vi "Database.vi"() -> ()   [LabVIEW 2017]
uses:
  D:/source/VI/JAC_Database/JAC_DataBase.dll
  JAC_DataBase.dll
panel:
  in  "筛选页数":i32=1 caption="页数" min=1 max=1 step=1 format="%.0f/1"
  in  "每页数量":i32
  in  "筛选按钮":bool
  in  "筛选值（支持模糊筛选）":string
  in  "表字段下拉菜单":u16(ring) caption="选择筛选字段"
  in  "表名下拉菜单":u16(ring) caption="选择数据表" items=["请选择...", "四轮定位工位配置", "大灯工位配置", "侧滑工位配置", "制动工位配置", "车辆信息表"]
  in  "删除按钮":bool
  in  "刷新按钮":bool caption="刷新显示"
  in  "修改按钮":bool caption="修改数据库"
  in  "页数":i32=1 min=0 max=1 step=1 format="%.0f/0"
  in  "停止按钮":bool
  in  "记录表格":string[][](table) caption="查询记录"
  # "说明：\n1、表记录的列首为数据库字段名，不可更改。\n2、表记录的行首为记录ID号，也不可更改。\n3、修改数据库以选择行（红色框）为修改范围，\n     选择有ID的记录为更新，无ID的记录为插入。\n4、删除记录，以选择行（红色框）为删除范围。"
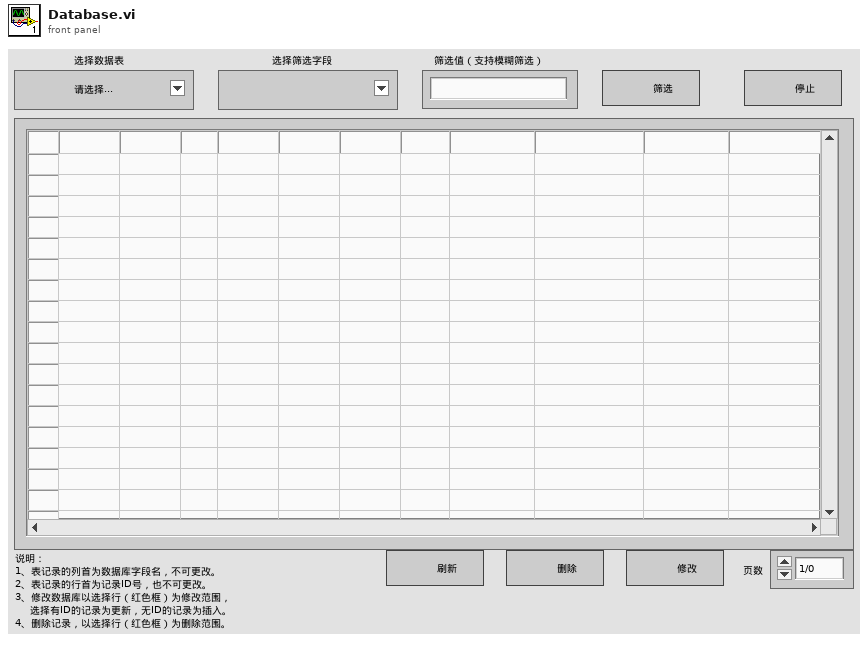
[diagram p1: front panel]
types:
  T1 = typedef "LVRowAndColumnTypeDef.ctl" = cluster{"Row":i32, "Column":i32}
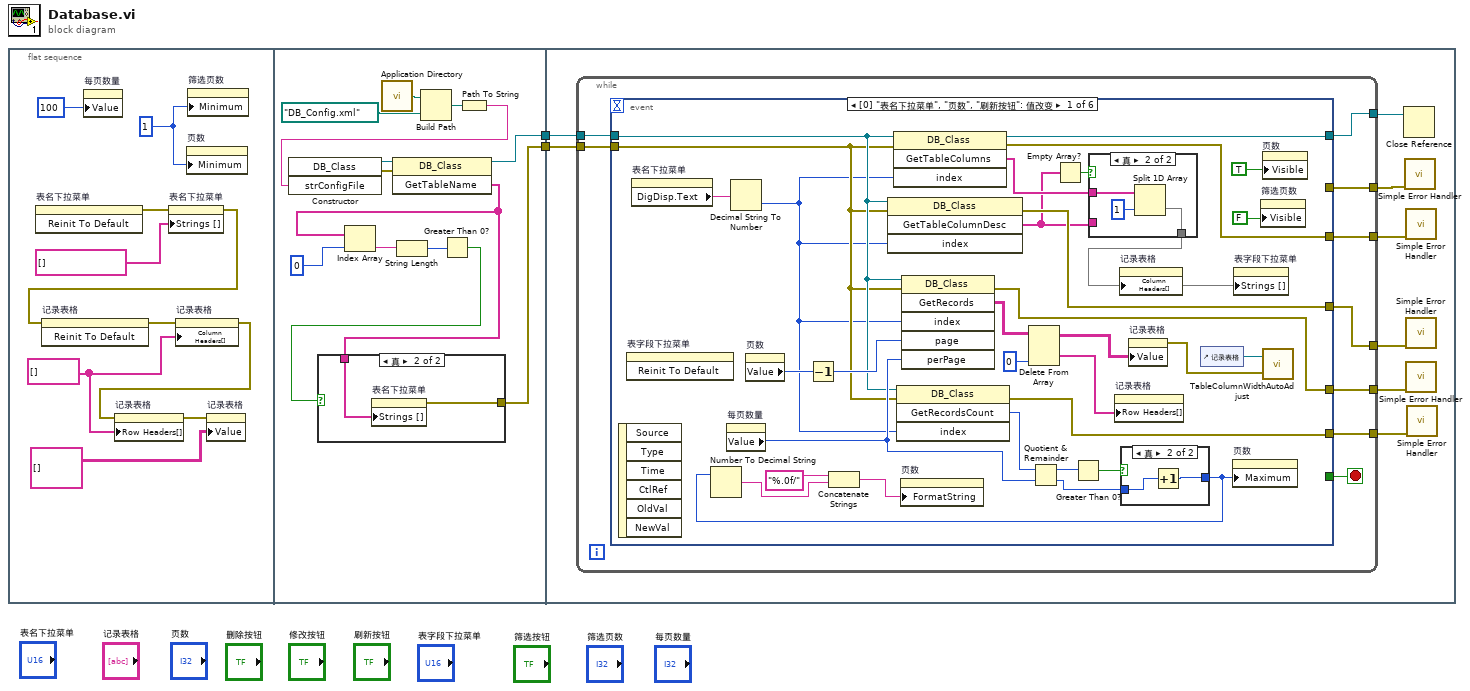
[diagram p0: block diagram]
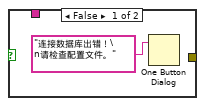
[diagram p2: hidden frame]
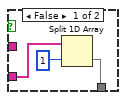
[diagram p3: hidden frame]
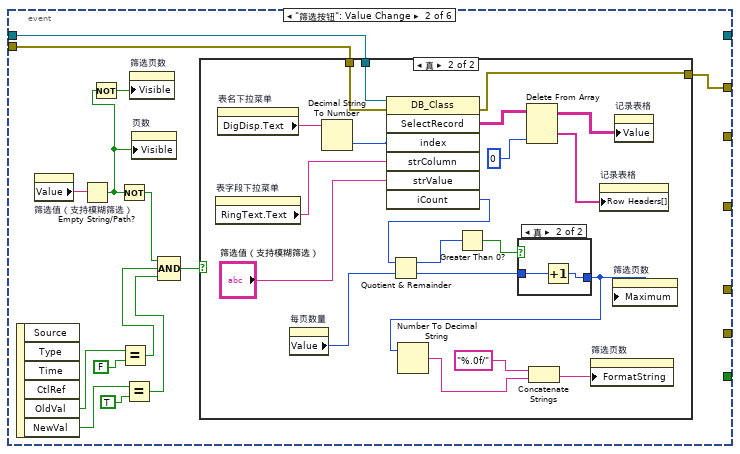
[diagram p5: hidden frame]
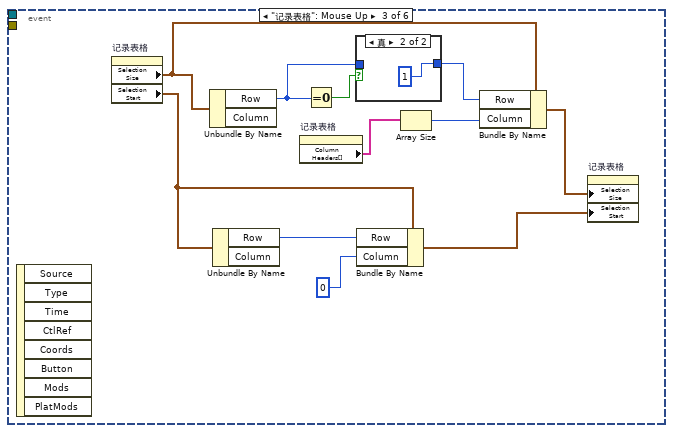
[diagram p8: hidden frame]
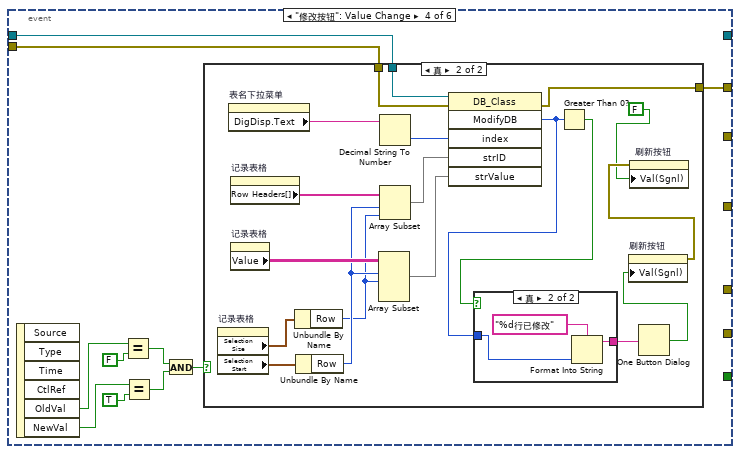
[diagram p10: hidden frame]
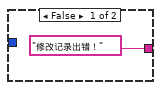
[diagram p12: hidden frame]
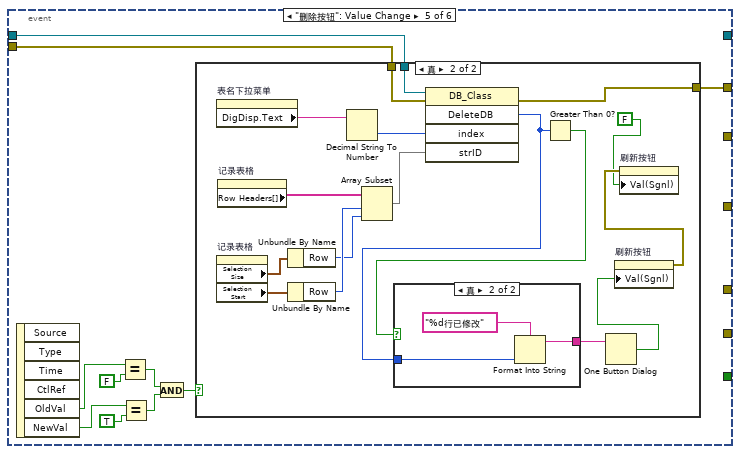
[diagram p13: hidden frame]
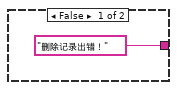
[diagram p15: hidden frame]
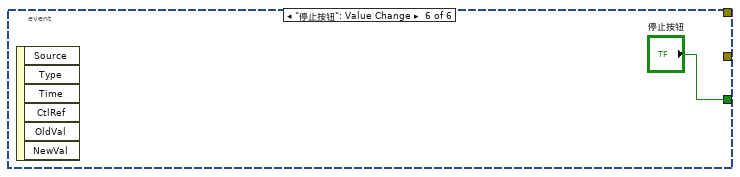
[diagram p16: hidden frame]
diagram:
  n1 = flat-sequence {
    tunnel: [w14] -> w2
    tunnel: [w13] -> w1
    tunnel: w2 -> [w33]
    tunnel: w1 -> [w32]
    frame #0 {
      w3 = 1
      w7 = string[] []
      n2 = invoke on="表名下拉菜单" class="Ring (严格)" method="Reinit To Default"() -> (error out=w12:errorcluster)  [unwired: 3 in, 2 out]
      n3 = property on="每页数量" class="DigNum (严格)"("Value"=100) -> ()  [unwired: 2 in, 2 out]
      n4 = property on="表名下拉菜单" class="Ring (严格)"(error in=w12, "Strings []"=string[] []) -> (error out=w10:errorcluster)  [unwired: 1 in, 1 out]
      n5 = invoke on="记录表格" class="Tbl (严格)" method="Reinit To Default"(error in=w10) -> (error out=w9:errorcluster)  [unwired: 2 in, 2 out]
      n6 = property on="记录表格" class="Tbl (严格)"(error in=w9, "Column Headers[]"=w7) -> (error out=w8:errorcluster)  [unwired: 1 in, 1 out]
      n7 = property on="记录表格" class="Tbl (严格)"(error in=w8, "Row Headers[]"=w7) -> (error out=w6:errorcluster)  [unwired: 1 in, 1 out]
      n8 = property on="页数" class="DigNum (严格)"("Minimum"=w3) -> ()  [unwired: 2 in, 2 out]
      n9 = property on="筛选页数" class="DigNum (严格)"("Minimum"=w3) -> ()  [unwired: 2 in, 2 out]
      n10 = property on="记录表格" class="Tbl (严格)"(error in=w6, "Value"=string[][] []) -> ()  [unwired: 1 in, 2 out]
    }
    frame #1 {
      n11 = call <vilib>:"Application Directory.vi"() -> ("Application Directory"=w17:path)
      n12 = Build Path(base path=w17, name or relative path=path "DB_Config.xml") -> (appended path=w18:path)
      n13 = Path To String(path=w18) -> (string=w19:string)
      n14 = constructor class="DB_Class"("strConfigFile"=w19) -> (reference out=w20:refnum<k24>, error out=w21:errorcluster)  [unwired: 3 in, 2 out]
      n15 = invoke on="调用节点" class="DB_Class" method="GetTableName"(reference=w20, error in=w21) -> (reference out=w14:refnum<k24>, "GetTableName"=w25:string[])  [unwired: 1 in, 1 out]
      n16 = Index Array(array=w25, index=0) -> (element=w22:string)
      n17 = String Length(string=w22) -> (length=w23:i32)
      n18 = Greater Than 0?(x=w23) -> (x > 0?=w24:bool)
      n19 = case shown="真" w24 {
        tunnel: w25 -> [_ w28]
        tunnel: [_ w27] -> w13
        frame False {
          n20 = One Button Dialog(message="连接数据库出错！\n请检查配置文件。") -> ()  [unwired: 1 in, 1 out]
        }
        frame True {
          n21 = property on="表名下拉菜单" class="Ring (严格)"("Strings []"=w28) -> (error out=w27:errorcluster)  [unwired: 2 in, 1 out]
        }
      }
    }
    frame #2 {
      n22 = while {
        tunnel: [w44] -> w36
        tunnel: [w43] -> w35
        tunnel: [w42] -> w34
        tunnel: w33 -> [w41]
        tunnel: w32 -> [w40]
        tunnel: [w39] -> w31
        tunnel: [w38] -> w30
        tunnel: [w37] -> w29
        stop <- w45 stop-if-true
        n23 = event shown="[0] \"表名下拉菜单\", \"页数\", \"刷新按钮\": 值改变" {
          selector: _ -> [_ _ _ _ _ _]
          dyn-events: _ -> [_ _ _ _ _ _]
          timeout: _ -> [_ _ _ _ _ _]
          tunnel: [_ _ _ _ _ "停止按钮"] -> w45
          tunnel: w41 -> [w56 w96 _ w140 w172 _]
          tunnel: w40 -> [w55 w95 _ w139 w171 _]
          tunnel: [w73 _ _ _ _ _] -> w44
          tunnel: [w72 _ _ _ _ _] -> w43
          tunnel: [_ w94 _ w138 w170 _] -> w42
          tunnel: [w71 _ _ _ _ _] -> w39
          tunnel: [w61 _ _ _ _ _] -> w38
          tunnel: [w52 _ _ _ _ _] -> w37
          event "表名下拉菜单", "页数", "刷新按钮": Value Change {
            n24 = event-data() -> ()  [unwired: 1 in, 6 out]
            n25 = invoke on="表字段下拉菜单" class="Ring (严格)" method="Reinit To Default"() -> ()  [unwired: 3 in, 3 out]
            n26 = property on="表名下拉菜单" class="Ring (严格)"() -> ("DigDisp.Text"=w49:string)  [unwired: 2 in, 2 out]
            n27 = property on="每页数量" class="DigNum (严格)"() -> ("Value"=w57:i32)  [unwired: 2 in, 2 out]
            n28 = Decimal String To Number(string=w49) -> (number=w48:i32)  [unwired: 2 in, 1 out]
            n29 = property on="页数" class="DigNum (严格)"() -> ("Value"=w58:i32)  [unwired: 2 in, 2 out]
            n30 = Decrement(x=w58) -> (x-1=w77:i32)
            n31 = invoke on="调用节点" class="DB_Class" method="GetTableColumnDesc"(reference=w56, error in=w55, "index"=w48) -> (error out=w52:errorcluster, "GetTableColumnDesc"=w51:string[])  [unwired: 1 in, 2 out]
            n32 = invoke class="DB_Class" method="GetTableColumns"(reference=w56, error in=w55, "index"=w48) -> (reference out=w61:refnum<k24>, error out=w73:errorcluster, "GetTableColumns"=w53:string[])  [unwired: 1 in, 1 out]
            n33 = invoke on="调用节点" class="DB_Class" method="GetRecordsCount"(reference=w56, error in=w55, "index"=w48) -> (error out=w71:errorcluster, "GetRecordsCount"=w67:i32)  [unwired: 1 in, 2 out]
            n34 = invoke class="DB_Class" method="GetRecords"(reference=w56, error in=w55, "index"=w48, "page"=w77, "perPage"=w57) -> (error out=w72:errorcluster, "GetRecords"=w76:string[][])  [unwired: 1 in, 4 out]
            n35 = Delete From Array(array=w76, index (col)=0) -> (deleted portion=w62:string[], array with subset deleted=w74:string[][])  [unwired: 2 in]
            n36 = Quotient & Remainder(x=w67, y=w57) -> (x-y*floor(x/y)=w70:i32, floor(x/y)=w68:i32)
            n37 = Empty Array?(array=w51) -> (empty?=w54:bool)
            n38 = Greater Than 0?(x=w70) -> (x > 0?=w69:bool)
            n39 = case shown="真" w54 {
              tunnel: w53 -> [_ w83]
              tunnel: [w78 w81] -> w50
              tunnel: w51 -> [w79 _]
              frame False {
                n40 = Split 1D Array(array=w79, index=1) -> (second subarray=w78:string[])  [unwired: 1 out]
              }
              frame True {
                n41 = Split 1D Array(array=w83, index=1) -> (second subarray=w81:string[])  [unwired: 1 out]
              }
            }
            n42 = property on="记录表格" class="Tbl (严格)"("Row Headers[]"=w62) -> ()  [unwired: 2 in, 2 out]
            n43 = property on="记录表格" class="Tbl (严格)"("Column Headers[]"=w50) -> ()  [unwired: 2 in, 2 out]
            n44 = case shown="真" w69 {
              tunnel: w68 -> [w84 w86]
              tunnel: [w84 w85] -> w63
              frame False {
              }
              frame True {
                n45 = Increment(x=w86) -> (x+1=w85:i32)
              }
            }
            n46 = Number To Decimal String(number=w63) -> (decimal integer string=w65:string)  [unwired: 1 in]
            n47 = Concatenate Strings("%.0f/", w65) -> (w64:string)
            n48 = property on="页数" class="DigNum (严格)"("FormatString"=w64) -> ()  [unwired: 2 in, 2 out]
            n49 = property on="记录表格" class="Tbl (严格)"("Value"=w74) -> (error out=w46:errorcluster)  [unwired: 2 in, 1 out]
            n50 = control-ref of="记录表格"() -> (w47:refnum<vi>)
            n51 = property on="页数" class="DigNum (严格)"("Maximum"=w63) -> ()  [unwired: 2 in, 2 out]
            n52 = property on="表字段下拉菜单" class="Ring (严格)"("Strings []"=w50) -> ()  [unwired: 2 in, 2 out]
            n53 = property on="筛选页数" class="DigNum (严格)"("Visible"=FALSE) -> ()  [unwired: 2 in, 2 out]
            n54 = property on="页数" class="DigNum (严格)"("Visible"=TRUE) -> ()  [unwired: 2 in, 2 out]
            n55 = call "TableColumnWidthAutoAdjust.vi"("错误输入"=w46, "Table输入"=w47) -> ()  [unwired: 2 out]
          }
          event "筛选按钮": Value Change {
            n56 = event-data() -> ("OldVal"=w100:bool, "NewVal"=w98:bool)  [unwired: 1 in, 4 out]
            n57 = property on="筛选值（支持模糊筛选）" class="Str"() -> ("Value"=w93:string)  [unwired: 2 in, 2 out]
            n58 = Empty String/Path?(string/path=w93) -> (empty?=w87:bool)
            n59 = Not(x=w87) -> (.not. x?=w88:bool)
            n60 = Not(x=w87) -> (.not. x?=w92:bool)
            n61 = Equal?(x=w100, y=FALSE) -> (x = y?=w91:bool)
            n62 = Equal?(x=w98, y=TRUE) -> (x = y?=w90:bool)
            n63 = property on="筛选页数" class="DigNum (严格)"("Visible"=w88) -> ()  [unwired: 2 in, 2 out]
            n64 = property on="页数" class="DigNum (严格)"("Visible"=w87) -> ()  [unwired: 2 in, 2 out]
            n65 = Compound Arithmetic op=AND ("复合运算")(w92, w91, w90) -> (w89:bool)
            n66 = case shown="真" w89 {
              tunnel: w96 -> [_ w120]
              tunnel: w95 -> [_ w119]
              tunnel: [_ w116] -> w94
              frame False {
              }
              frame True {
                n67 = property on="表字段下拉菜单" class="Ring (严格)"() -> ("RingText.Text"=w118:string)  [unwired: 2 in, 2 out]
                n68 = property on="表名下拉菜单" class="Ring (严格)"() -> ("DigDisp.Text"=w101:string)  [unwired: 2 in, 2 out]
                n69 = property on="每页数量" class="DigNum (严格)"() -> ("Value"=w103:i32)  [unwired: 2 in, 2 out]
                n70 = Decimal String To Number(string=w101) -> (number=w102:i32)  [unwired: 2 in, 1 out]
                n71 = invoke on="调用节点" class="DB_Class" method="SelectRecord"(reference=w120, error in=w119, "index"=w102, "strColumn"=w118, "strValue"="筛选值（支持模糊筛选）") -> (error out=w116:errorcluster, "SelectRecord"=w115:string[][], "iCount"=w110:i32)  [unwired: 2 in, 4 out]
                n72 = Quotient & Remainder(x=w110, y=w103) -> (x-y*floor(x/y)=w111:i32, floor(x/y)=w108:i32)
                n73 = Greater Than 0?(x=w111) -> (x > 0?=w109:bool)
                n74 = case shown="真" w109 {
                  tunnel: w108 -> [w121 w123]
                  tunnel: [w121 w122] -> w105
                  frame False {
                  }
                  frame True {
                    n75 = Increment(x=w123) -> (x+1=w122:i32)
                  }
                }
                n76 = Number To Decimal String(number=w105) -> (decimal integer string=w107:string)  [unwired: 1 in]
                n77 = Delete From Array(array=w115, index (col)=0) -> (deleted portion=w112:string[], array with subset deleted=w113:string[][])  [unwired: 2 in]
                n78 = Concatenate Strings("%.0f/", w107) -> (w104:string)
                n79 = property on="筛选页数" class="DigNum (严格)"("FormatString"=w104) -> ()  [unwired: 2 in, 2 out]
                n80 = property on="记录表格" class="Tbl (严格)"("Row Headers[]"=w112) -> ()  [unwired: 2 in, 2 out]
                n81 = property on="筛选页数" class="DigNum (严格)"("Maximum"=w105) -> ()  [unwired: 2 in, 2 out]
                n82 = property on="记录表格" class="Tbl (严格)"("Value"=w113) -> ()  [unwired: 2 in, 2 out]
              }
            }
          }
          event "记录表格": Mouse Up {
            n83 = event-data() -> ()  [unwired: 1 in, 8 out]
            n84 = property on="记录表格" class="Tbl (严格)"() -> ("Selection Size"=w134:T1, "Selection Start"=w127:T1)  [unwired: 2 in, 2 out]
            n85 = Unbundle By Name(w134) -> ("Row"=w130:i32)  [unwired: 1 out]
            n86 = Unbundle By Name(w127) -> ("Row"=w124:i32)  [unwired: 1 out]
            n87 = property on="记录表格" class="Tbl (严格)"() -> ("Column Headers[]"=w129:string[])  [unwired: 2 in, 2 out]
            n88 = Equal To 0?(x=w130) -> (x = 0?=w131:bool)
            n89 = case shown="真" w131 {
              tunnel: [w135 1] -> w133
              tunnel: w130 -> [w135 _]
              frame False {
              }
              frame True {
              }
            }
            n90 = Bundle By Name(cluster=w127, "Row"=w124, "Column"=0) -> (w126:T1)
            n91 = Array Size(array=w129) -> (size(s)=w128:i32)
            n92 = Bundle By Name(cluster=w134, "Row"=w133, "Column"=w128) -> (w132:T1)
            n93 = property on="记录表格" class="Tbl (严格)"("Selection Size"=w132, "Selection Start"=w126) -> ()  [unwired: 2 in, 2 out]
          }
          event "修改按钮": Value Change {
            n94 = event-data() -> ("OldVal"=w137:bool, "NewVal"=w145:bool)  [unwired: 1 in, 4 out]
            n95 = Equal?(x=w137, y=FALSE) -> (x = y?=w143:bool)
            n96 = Equal?(x=w145, y=TRUE) -> (x = y?=w142:bool)
            n97 = And(x=w143, y=w142) -> (x .and. y?=w141:bool)
            n98 = case shown="真" w141 {
              tunnel: w140 -> [_ w159]
              tunnel: w139 -> [_ w158]
              tunnel: [_ w152] -> w138
              frame False {
              }
              frame True {
                n99 = property on="记录表格" class="Tbl (严格)"() -> ("Selection Size"=w164:T1, "Selection Start"=w165:T1)  [unwired: 2 in, 2 out]
                n100 = property on="表名下拉菜单" class="Ring (严格)"() -> ("DigDisp.Text"=w148:string)  [unwired: 2 in, 2 out]
                n101 = property on="记录表格" class="Tbl (严格)"() -> ("Row Headers[]"=w163:string[])  [unwired: 2 in, 2 out]
                n102 = property on="记录表格" class="Tbl (严格)"() -> ("Value"=w162:string[][])  [unwired: 2 in, 2 out]
                n103 = Unbundle By Name(w164) -> ("Row"=w160:i32)
                n104 = Unbundle By Name(w165) -> ("Row"=w161:i32)
                n105 = Array Subset(array=w162, index (row)=w161, length (row)=w160) -> (w156:string[][])  [unwired: 2 in]
                n106 = Decimal String To Number(string=w148) -> (number=w147:i32)  [unwired: 2 in, 1 out]
                n107 = Array Subset(array=w163, index=w161, length=w160) -> (w157:string[])
                n108 = invoke on="调用节点" class="DB_Class" method="ModifyDB"(reference=w159, error in=w158, "index"=w147, "strID"=w157, "strValue"=w156) -> (error out=w152:errorcluster, "ModifyDB"=w154:i32)  [unwired: 1 in, 4 out]
                n109 = Greater Than 0?(x=w154) -> (x > 0?=w155:bool)
                n110 = case shown="真" w155 {
                  tunnel: w154 -> [_ w168]
                  tunnel: ["修改记录出错！" w167] -> w153
                  frame False {
                  }
                  frame True {
                    n111 = Format Into String(format string="%d行已修改", w168) -> (resulting string=w167:string)  [unwired: 2 in, 1 out]
                  }
                }
                n112 = One Button Dialog(message=w153) -> (true=w151:bool)  [unwired: 1 in]
                n113 = property on="刷新按钮" class="Bool (严格)"("Val(Sgnl)"=w151) -> (error out=w150:errorcluster)  [unwired: 2 in, 1 out]
                n114 = property on="刷新按钮" class="Bool (严格)"(error in=w150, "Val(Sgnl)"=FALSE) -> ()  [unwired: 1 in, 2 out]
              }
            }
          }
          event "删除按钮": Value Change {
            n115 = event-data() -> ("OldVal"=w175:bool, "NewVal"=w174:bool)  [unwired: 1 in, 4 out]
            n116 = Equal?(x=w175, y=FALSE) -> (x = y?=w177:bool)
            n117 = Equal?(x=w174, y=TRUE) -> (x = y?=w176:bool)
            n118 = And(x=w177, y=w176) -> (x .and. y?=w173:bool)
            n119 = case shown="真" w173 {
              tunnel: w172 -> [_ w196]
              tunnel: w171 -> [_ w195]
              tunnel: [_ w194] -> w170
              frame False {
              }
              frame True {
                n120 = property on="表名下拉菜单" class="Ring (严格)"() -> ("DigDisp.Text"=w181:string)  [unwired: 2 in, 2 out]
                n121 = property on="记录表格" class="Tbl (严格)"() -> ("Selection Size"=w193:T1, "Selection Start"=w192:T1)  [unwired: 2 in, 2 out]
                n122 = property on="记录表格" class="Tbl (严格)"() -> ("Row Headers[]"=w191:string[])  [unwired: 2 in, 2 out]
                n123 = Unbundle By Name(w193) -> ("Row"=w189:i32)
                n124 = Unbundle By Name(w192) -> ("Row"=w190:i32)
                n125 = Decimal String To Number(string=w181) -> (number=w180:i32)  [unwired: 2 in, 1 out]
                n126 = Array Subset(array=w191, index=w190, length=w189) -> (w188:string[])
                n127 = invoke on="调用节点" class="DB_Class" method="DeleteDB"(reference=w196, error in=w195, "index"=w180, "strID"=w188) -> (error out=w194:errorcluster, "DeleteDB"=w186:i32)  [unwired: 1 in, 3 out]
                n128 = Greater Than 0?(x=w186) -> (x > 0?=w187:bool)
                n129 = case shown="真" w187 {
                  tunnel: w186 -> [_ w199]
                  tunnel: ["删除记录出错！" w198] -> w185
                  frame False {
                  }
                  frame True {
                    n130 = Format Into String(format string="%d行已修改", w199) -> (resulting string=w198:string)  [unwired: 2 in, 1 out]
                  }
                }
                n131 = One Button Dialog(message=w185) -> (true=w184:bool)  [unwired: 1 in]
                n132 = property on="刷新按钮" class="Bool (严格)"("Val(Sgnl)"=w184) -> (error out=w183:errorcluster)  [unwired: 2 in, 1 out]
                n133 = property on="刷新按钮" class="Bool (严格)"(error in=w183, "Val(Sgnl)"=FALSE) -> ()  [unwired: 1 in, 2 out]
              }
            }
          }
          event "停止按钮": Value Change {
            n134 = event-data() -> ()  [unwired: 1 in, 6 out]
          }
        }
      }
      n135 = Close Reference(reference=w30) -> ()  [unwired: 1 in, 1 out]
      n136 = call <vilib>:"Simple Error Handler.vi"("error in (no error)"=w34) -> ()  [unwired: 4 in, 5 out]
      n137 = call <vilib>:"Simple Error Handler.vi"("error in (no error)"=w36) -> ()  [unwired: 4 in, 5 out]
      n138 = call <vilib>:"Simple Error Handler.vi"("error in (no error)"=w29) -> ()  [unwired: 4 in, 5 out]
      n139 = call <vilib>:"Simple Error Handler.vi"("error in (no error)"=w35) -> ()  [unwired: 4 in, 5 out]
      n140 = call <vilib>:"Simple Error Handler.vi"("error in (no error)"=w31) -> ()  [unwired: 4 in, 5 out]
    }
  }
